vi "TDMSErrorTets.vi"() -> ()   [LabVIEW 2012]
uses:
  Oscilloscope/TypeDefs/DataTypes/Data.ctl
  Oscilloscope/TypeDefs/DataTypes/DAQConfig.ctl
  Oscilloscope/TypeDefs/DataTypes/Acquisition.ctl
  Oscilloscope/TypeDefs/DataTypes/Current.ctl
  Oscilloscope/TypeDefs/DataTypes/StopCondition.ctl
  Oscilloscope/TypeDefs/DataTypes/Measurement.ctl
  Oscilloscope/TypeDefs/DataTypes/UIReferences.ctl
  Oscilloscope/TypeDefs/DataTypes/RunInfo.ctl
  TypeDefs/DataTypes/SystemStatus.ctl
panel:
  in  "Data In":T1={"DAQ Config Data"={"Vertical"={"Coupling"=1, "Offset (V)"=-0.5, "Range (V)"=2.0, "Impedance"=50.0}, "Horizontal"={"Offset Time"=0.0, "Sample Time (S)"=22.0, "Sample Points"=1000}, "Trigger\n"={"Lower Level (V)"=-0.02, "Trigger Slope"=1, "Trigger Source"=10}, "Acquisition"={"Trigger Mode"=1, "Initiate Continuously"=0, "Acquire Type"=0, "Acquire Count"=1}, "Channel"=0, "Instrument Handle"=0, "Error"={"status"=FALSE, "code"=0, "source"=""}, "State"=1}, "Acquisition"={"Current"={"Acquiring Now?"=FALSE, "Waveforms Acquired"=0.0, "Start of Acquisition"=timestamp(0 s since 1904-01-01), "Acquisition Name"=""}, "Stop Condition"={"Quota"=3000.0, "Duration (S)"=22, "Stop Condition"=FALSE}, "Config Needed"=FALSE}, "Measurement"={"Waveform"={"t0"=timestamp(0 s since 1904-01-01), "dt"=1.0, "Y"=[]}, "Peak Heights"=[], "Acquisition Time"=timestamp(0 s since 1904-01-01), "File Path"=path "C:/Users/lab-341/Desktop/Reed/Oscilloscope VI/pulses.tdms", "TDMS File Handle"=refnum}, "UI References"={"Acquire"=refnum, "Configure DAQ"=refnum, "Measurement (Ch1)"=refnum, "Update Needed?"=FALSE, "New Run"=refnum, "Signal"=refnum}, "Run Info"={"Active Run?"=FALSE, "Run Notes"="Enter in notes explaining the purpose of the run and any unusual steps taken in the process. This should make it clear why the data was taken. e.g. \"Measuring LXe scintillation light with Teflon\" or \"Measuring dark pulses to determine SPE gain.\" Concise is good but precise is better.", "User Name"="", "Campaign ID#"="", "Run Name"="", "Start Time"=timestamp(0 s since 1904-01-01), "End Time"=timestamp(0 s since 1904-01-01)}, "System Status"={"Bias Voltage"=0.0, "SiPM Temperature"=[], "Slow Control User"="", "LXe"=0.0}, "Acquisition Info"={"Trigger Mode"=FALSE, "Acquisition Mode"=FALSE, "Bias Voltage (V)"=0.0, "Preamplifier"=0, "Shaping Amplifier"=0, "Acquisition Notes"="", "1"=FALSE, "2"=FALSE}} {"Acquisition Info"."Shaping Amplifier" items=["CR-200-100ns", "CR-200-1us"]; "Acquisition Info"."Preamplifier" items=["CR-Z-113-1k", "CR-Z-113-5k", "CR-Z-SiPM"]; "DAQ Config Data"."State" items=["Enable"=1, "Disable"=0]; "DAQ Config Data"."Channel" items=["Input Channel 1", "Input Channel 2", "Input Channel 3", "Input Channel 4"]; "DAQ Config Data"."Acquisition"."Acquire Type" items=["Normal"=0, "Average"=1, "Envelope"=2, "Peak Detect"=3, "High Resolution"=4, "Fast"=5, "Equivalent Time"=16]; "DAQ Config Data"."Acquisition"."Initiate Continuously" items=["Continuously"=1, "Single Capture"=0]; "DAQ Config Data"."Acquisition"."Trigger Mode" items=["Auto", "Normal"]; "DAQ Config Data"."Trigger"."Trigger Source" items=["TTL0", "TTL1", "TTL2", "TTL3", "TTL4", "TTL5", "TTL6", "TTL7", "ECL0", "ECL1", "Input Channel 1", "Input Channel 2", "Input Channel 3", "Input Channel 4", "External Trigger Source", "STAR", "Manual Trigger", "Pattern"]; "DAQ Config Data"."Trigger"."Trigger Slope" items=["Rising Edge", "Falling Edge"]; "DAQ Config Data"."Horizontal"."Sample Time (S)" items=["0.5"=0.5, "0.4"=0.4, "0.25"=0.25, "0.2"=0.2, "0.1"=0.1, "0.05"=0.05, "0.04"=0.04, "0.025"=0.025, "0.02"=0.02, "0.01"=0.01, "0.005"=0.005, "0.004"=0.004, "0.0025"=0.0025, "0.002"=0.002, "0.001"=0.001, "5E-4"=0.0005, "4E-4"=0.0004, "2.5E-4"=0.00025, "2E-4"=0.0002, "1E-4"=0.0001, "5E-5"=5e-05, "4E-5"=4e-05, "2E-5"=2e-05, "5E-6"=5e-06, "1E-6"=1e-06, "5E-7"=5e-07, "1E-7"=1e-07, "5E-8"=5e-08, "1E-8"=1e-08]; "DAQ Config Data"."Vertical"."Impedance" items=["50 Ohm"=50.0, "1 MOhm"=1000000.0]; "DAQ Config Data"."Vertical"."Range (V)" items=["10"=10.0, "5"=5.0, "2"=2.0, "1"=1.0, "0.4"=0.4, "0.2"=0.2, "0.08"=0.08, "0.04"=0.04, "0.02"=0.02, "0.01"=0.01]; "DAQ Config Data"."Vertical"."Coupling" items=["AC", "DC"]}
  # "Shaper Gain"
  # "Self"
  # "Fast"
  # "Solicited"
  # "Standard"
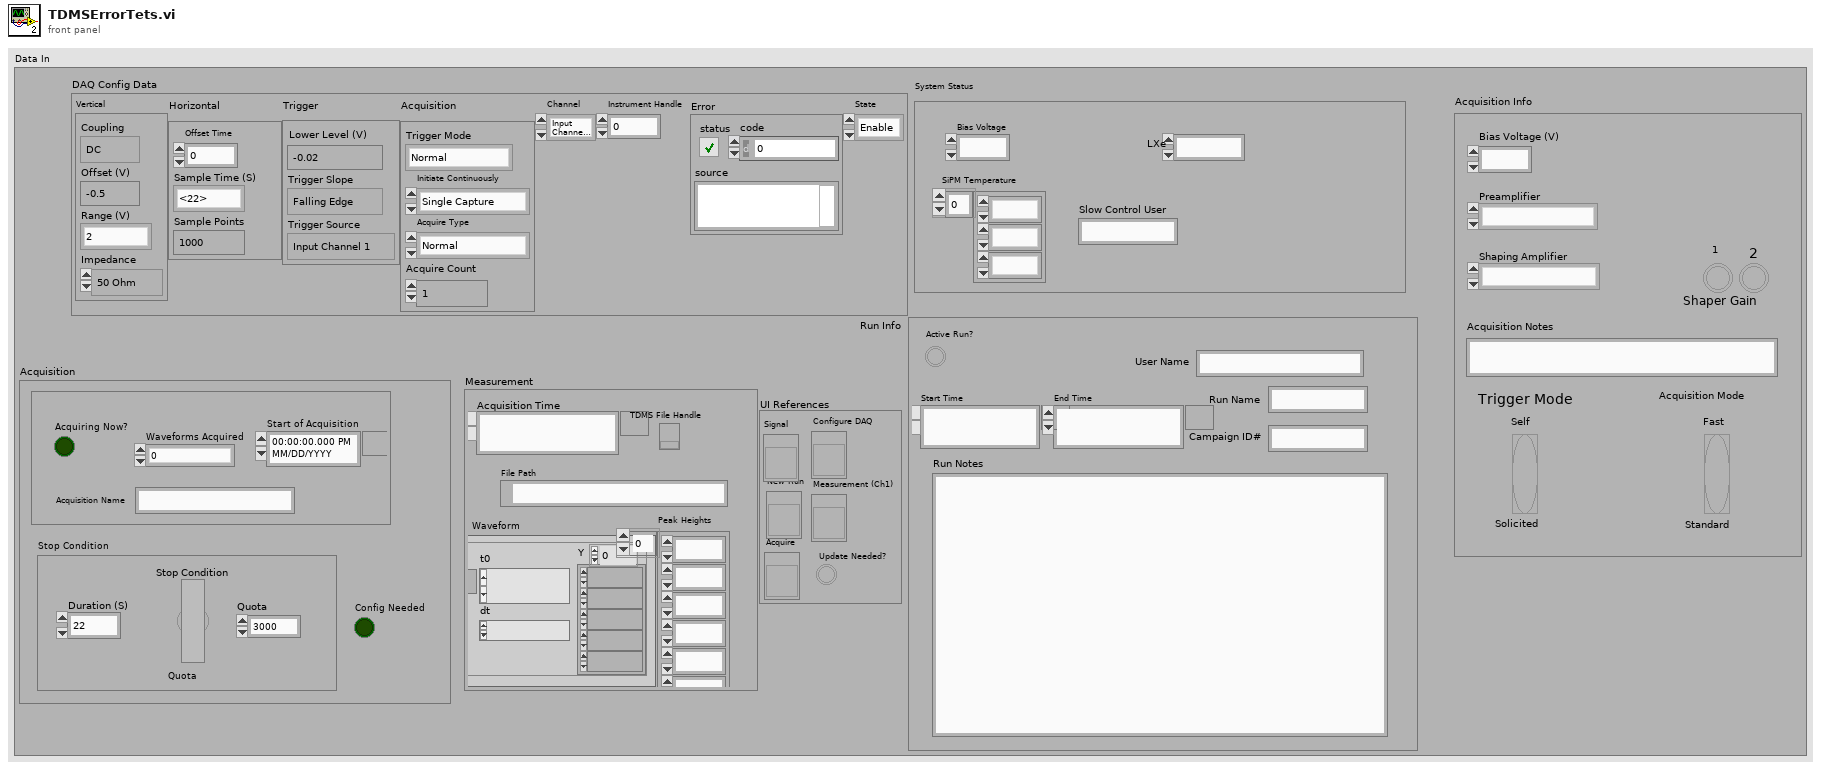
[diagram p1: front panel]
types:
  T1 = typedef "Data.ctl" = cluster{"DAQ Config Data":T2, "Acquisition":T3, "Measurement":T6, "UI References":T7, "Run Info":T8, "System Status":T9, "Acquisition Info":cluster{"Trigger Mode":bool, "Acquisition Mode":bool, "Bias Voltage (V)":dbl, "Preamplifier":u16, "Shaping Amplifier":u16, "Acquisition Notes":string, "1":bool, "2":bool}}
  T2 = typedef "DAQConfig.ctl" = cluster{"Vertical":cluster{"Coupling":i32, "Offset (V)":dbl, "Range (V)":dbl, "Impedance":dbl}, "Horizontal":cluster{"Offset Time":dbl, "Sample Time (S)":dbl, "Sample Points":u32}, "Trigger\n":cluster{"Lower Level (V)":dbl, "Trigger Slope":i32, "Trigger Source":i32}, "Acquisition":cluster{"Trigger Mode":i32, "Initiate Continuously":i32, "Acquire Type":i32, "Acquire Count":i32}, "Channel":i32, "Instrument Handle":i32, "Error":errorcluster, "State":i32}
  T3 = typedef "Acquisition.ctl" = cluster{"Current":T4, "Stop Condition":T5, "Config Needed":bool}
  T4 = typedef "Current.ctl" = cluster{"Acquiring Now?":bool, "Waveforms Acquired":dbl, "Start of Acquisition":timestamp, "Acquisition Name":string}
  T5 = typedef "StopCondition.ctl" = cluster{"Quota":dbl, "Duration (S)":u16, "Stop Condition":bool}
  T6 = typedef "Measurement.ctl" = cluster{"Waveform":waveform(dbl), "Peak Heights":dbl[], "Acquisition Time":timestamp, "File Path":path, "TDMS File Handle":refnum<k34>}
  T7 = typedef "UIReferences.ctl" = cluster{"Acquire":refnum<vi>, "Configure DAQ":refnum<vi>, "Measurement (Ch1)":refnum<vi>, "Update Needed?":bool, "New Run":refnum<vi>, "Signal":refnum<vi>}
  T8 = typedef "RunInfo.ctl" = cluster{"Active Run?":bool, "Run Notes":string, "User Name":string, "Campaign ID#":string, "Run Name":string, "Start Time":timestamp, "End Time":timestamp}
  T9 = typedef "SystemStatus.ctl" = cluster{"Bias Voltage":dbl, "SiPM Temperature":dbl[], "Slow Control User":string, "LXe":dbl}
  T10 = enum16{"open", "open or create", "create or replace", "create", "open (read-only)"}
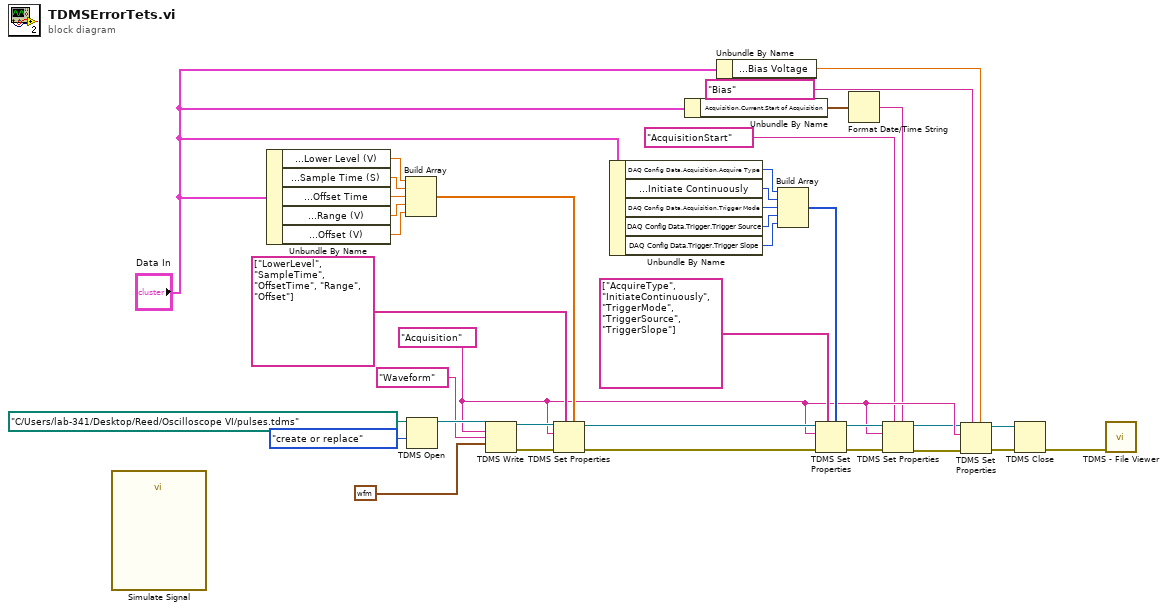
[diagram p0: block diagram]
diagram:
  w6 = "Acquisition" ("group name in (Untitled)")
  n1 = call "Simulate Signal"() -> ()  [unwired: 14 in, 2 out]
  n2 = Unbundle By Name("Data In") -> ("DAQ Config Data.Trigger.Lower Level (V)"=w30:dbl, "DAQ Config Data.Horizontal.Sample Time (S)"=w29:dbl, "DAQ Config Data.Horizontal.Offset Time"=w28:dbl, "DAQ Config Data.Vertical.Range (V)"=w27:dbl, "DAQ Config Data.Vertical.Offset (V)"=w26:dbl)
  n3 = Build Array(w30, w29, w28, w27, w26) -> (w25:dbl[])
  n4 = TDMS Open(10:T10."create or replace" ("operation (0:open)"), 11:path "C:/Users/lab-341/Desktop/Reed/Oscilloscope VI/pulses.tdms" ("file path")) -> (3:w37:refnum<k34>)  [unwired: 4 in, 1 out]
  n5 = TDMS Write(0:w37, 5:w6, 7:"Waveform" ("channel name(s) in (Untitled)"), 9:waveform(dbl) {"t0"=timestamp(3681306574.4557176 s since 1904-01-01), "dt"=0.022, "Y"=array[1000 elements]} ("Waveform")) -> (4:w32:refnum<k34>, 15:w31:errorcluster)  [unwired: 2 in, 2 out]
  n6 = TDMS Set Properties(5:w25, 7:string[] ["LowerLevel", "SampleTime", "OffsetTime", "Range", "Offset"] ("property names"), 8:w31, 10:w6, 11:w32) -> (0:w21:errorcluster, 3:w22:refnum<k34>)  [unwired: 1 in, 2 out]
  n7 = Unbundle By Name("Data In") -> ("DAQ Config Data.Acquisition.Acquire Type"=w20:i32, "DAQ Config Data.Acquisition.Initiate Continuously"=w19:i32, "DAQ Config Data.Acquisition.Trigger Mode"=w18:i32, "DAQ Config Data.Trigger.Trigger Source"=w17:i32, "DAQ Config Data.Trigger.Trigger Slope"=w16:i32)
  n8 = Unbundle By Name("Data In") -> ("Acquisition.Current.Start of Acquisition"=w2:timestamp)
  n9 = Unbundle By Name("Data In") -> ("System Status.Bias Voltage"=w12:dbl)
  n10 = Build Array(w20, w19, w18, w17, w16) -> (w15:i32[])
  n11 = TDMS Set Properties(5:w15, 7:string[] ["AcquireType", "InitiateContinuously", "TriggerMode", "TriggerSource", "TriggerSlope"] ("property names"), 8:w21, 10:w6, 11:w22) -> (0:w7:errorcluster, 3:w8:refnum<k34>)  [unwired: 1 in, 2 out]
  n12 = Format Date/Time String(seconds (now)=w2) -> (date/time string=w1:string)  [unwired: 2 in]
  n13 = TDMS Set Properties(5:w1, 7:"AcquisitionStart", 8:w7, 10:w6, 11:w8) -> (0:w4:errorcluster, 3:w5:refnum<k34>)  [unwired: 1 in, 2 out]
  n14 = TDMS Set Properties(5:w12, 7:"Bias", 8:w4, 10:w6, 11:w5) -> (0:w9:errorcluster, 3:w10:refnum<k34>)  [unwired: 1 in, 2 out]
  n15 = TDMS Close(8:w9, 11:w10) -> (0:w23:errorcluster)  [unwired: 1 out]
  n16 = call <vilib>:"TDMS - File Viewer.vi"("error in (no error)"=w23) -> ()  [unwired: 5 in, 2 out]
